vi "Retrieve WMI String.vi"(8 "error in":errorcluster, 9 "wmiProperty":string="SerialNumber", 10 "wmiClass":string="Win32_Bios", 11 "Scope":string="root\\cimv2") -> (0 "Error Out":errorcluster, 2 "Values":string[](array[string]), 3 "LastValue":string="D6N0CY261389233     ")   [LabVIEW 2013]
doc: "Retrieve a string value of a WMI property given a namespace (<b>Scope</b>), Class (<b>wmiClass</b>) and a property name (<b>wmiProperty</b>)."
uses:
  System.Management
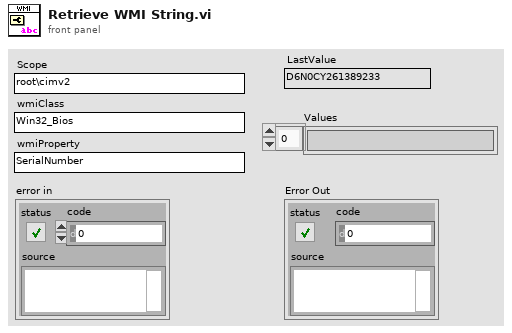
[diagram p1: front panel]
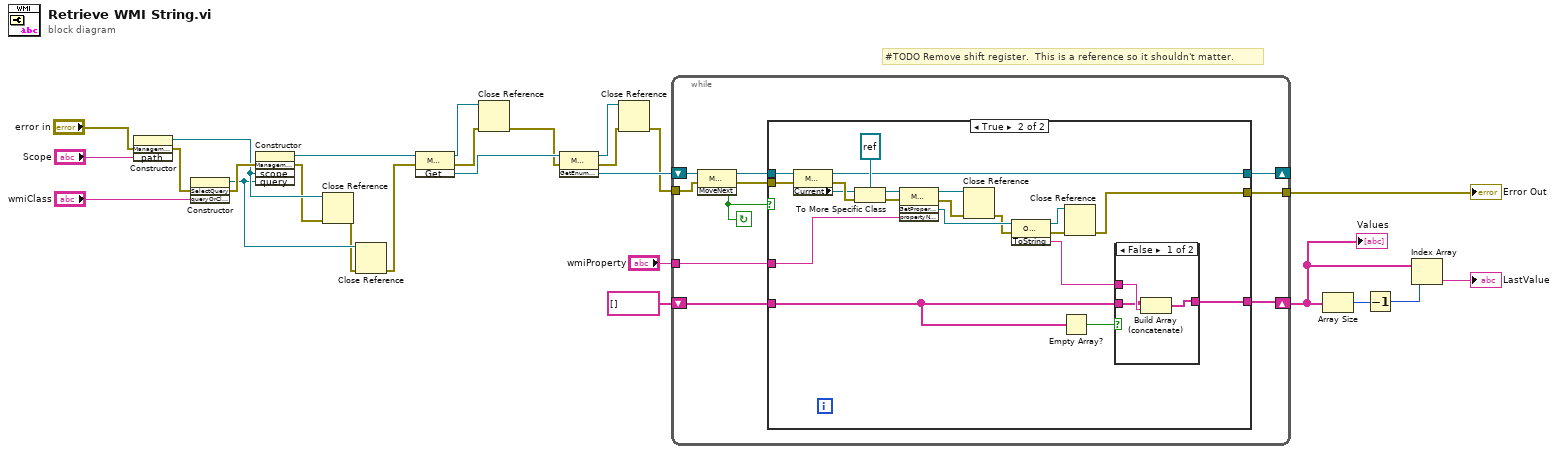
[diagram p0: block diagram]
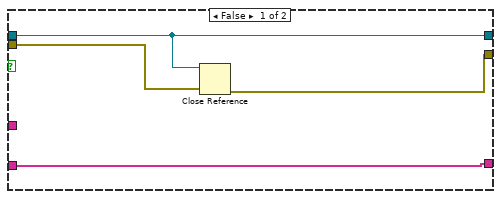
[diagram p2: hidden frame]
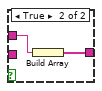
[diagram p3: hidden frame]
diagram:
  # "#TODO Remove shift register.  This is a reference so it shouldn't matter."
  n1 = constructor class="ManagementScope"(error in="error in", "path"="Scope") -> (reference out=w15:refnum<k24>, error out=w19:errorcluster)  [unwired: 2 in, 2 out]
  n2 = constructor class="SelectQuery"(error in=w19, "queryOrClassName"="wmiClass") -> (reference out=w13:refnum<k24>, error out=w18:errorcluster)  [unwired: 2 in, 2 out]
  n3 = constructor class="ManagementObjectSearcher"(error in=w18, "scope"=w15, "query"=w13) -> (reference out=w26:refnum<k24>, error out=w14:errorcluster)  [unwired: 2 in, 3 out]
  n4 = Close Reference(reference=w15, error in (no error)=w14) -> (error out=w12:errorcluster)
  n5 = Close Reference(reference=w13, error in (no error)=w12) -> (error out=w11:errorcluster)
  n6 = invoke class="ManagementObjectSearcher" method="Get"(reference=w26, error in=w11) -> (reference out=w22:refnum<k24>, error out=w4:errorcluster, "Get"=w25:refnum<k24>)  [unwired: 1 in]
  n7 = Close Reference(reference=w22, error in (no error)=w4) -> (error out=w3:errorcluster)
  n8 = invoke class="ManagementObjectCollection" method="GetEnumerator"(reference=w25, error in=w3) -> (reference out=w21:refnum<k24>, error out=w2:errorcluster, "GetEnumerator"=w20:refnum<k24>)  [unwired: 1 in]
  n9 = Close Reference(reference=w21, error in (no error)=w2) -> (error out=w1:errorcluster)
  n10 = while {
    shift-right: [w34] -> _
    shift-left: w20 -> [w36]
    tunnel: [w30] -> w9
    tunnel: w1 -> [w32]
    tunnel: "wmiProperty" -> [w31]
    shift-right: [w27] -> w6
    shift-left: string[] [] -> [w28]
    stop <- w29 continue-if-true
    n11 = invoke class="ManagementObjectCollection+Mana" method="MoveNext"(reference=w36, error in=w32) -> (reference out=w33:refnum<k24>, error out=w35:errorcluster, "MoveNext"=w29:bool)  [unwired: 1 in]
    n12 = case shown="True" w29 {
      tunnel: w35 -> [w38 w60]
      tunnel: [w39 w58] -> w34
      tunnel: w33 -> [w39 w55]
      tunnel: w31 -> [_ w45]
      tunnel: [w37 w49] -> w30
      tunnel: w28 -> [w40 w41]
      tunnel: [w40 w42] -> w27
      frame False {
        n13 = Close Reference(reference=w39, error in (no error)=w38) -> (error out=w37:errorcluster)
      }
      frame True {
        n14 = property class="ManagementObjectCollection+Mana"(reference=w55, error in=w60) -> (reference out=w58:refnum<k24>, error out=w57:errorcluster, "Current"=w56:refnum<k24>)
        n15 = To More Specific Class(target class=refnum<k24> refnum ("Current"), reference=w56, error in=w57) -> (specific class reference=w54:refnum<k24>, error out=w52:errorcluster)
        n16 = invoke class="ManagementObject" method="GetPropertyValue"(reference=w54, error in=w52, "propertyName"=w45) -> (reference out=w48:refnum<k24>, error out=w47:errorcluster, "GetPropertyValue"=w53:refnum<k24>)  [unwired: 1 in, 1 out]
        n17 = Close Reference(reference=w48, error in (no error)=w47) -> (error out=w46:errorcluster)
        n18 = invoke class="Object" method="ToString"(reference=w53, error in=w46) -> (reference out=w51:refnum<k24>, error out=w50:errorcluster, "ToString"=w43:string)  [unwired: 1 in]
        n19 = Empty Array?(array=w41) -> (empty?=w44:bool)
        n20 = Close Reference(reference=w51, error in (no error)=w50) -> (error out=w49:errorcluster)
        n21 = case shown="False" w44 {
          tunnel: w43 -> [w62 w65]
          tunnel: [w63 w64] -> w42
          tunnel: w41 -> [w61 _]
          frame False {
            n22 = Build Array (concatenate)(w61, w62) -> (w63:string[])
          }
          frame True {
            n23 = Build Array(w65) -> (w64:string[])
          }
        }
      }
    }
  }
  "Error Out" <- w9
  "Values" <- w6
  n24 = Array Size(array=w6) -> (size(s)=w8:i32)
  n25 = Decrement(x=w8) -> (x-1=w7:i32)
  n26 = Index Array(array=w6, index=w7) -> (element=→"LastValue":string)
